vi "temperatureFGV.vi"(4 "error in (no error)":errorcluster, 5 "InputFan":bool=TRUE, 6 "state":T1, 7 "InputTemp":dbl) -> (0 "error out":errorcluster, 1 "OutputFan":bool=TRUE, 3 "OutputTemp":dbl)   [LabVIEW 2024]
uses:
  statesFGV.ctl
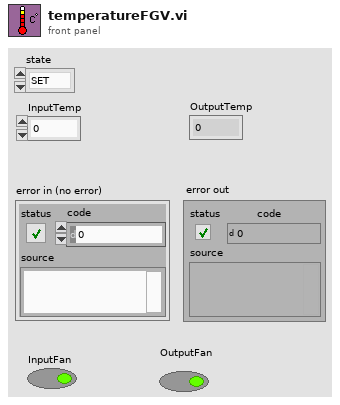
[diagram p1: front panel]
types:
  T1 = typedef "statesFGV.ctl" = enum16{"SET", "GET"}
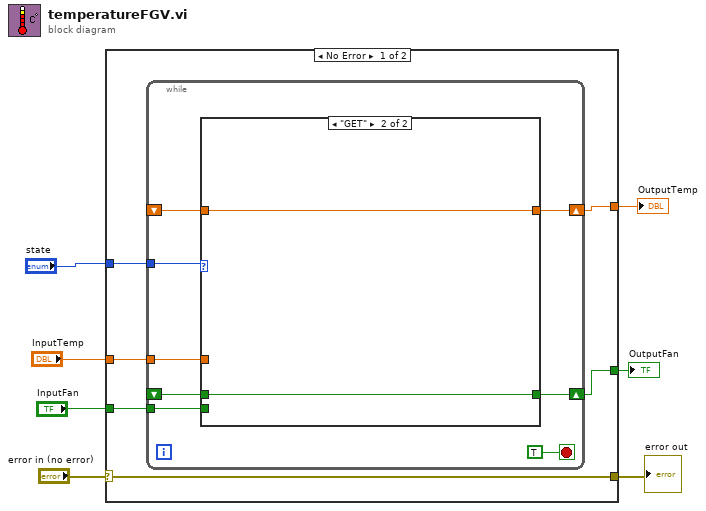
[diagram p0: block diagram]
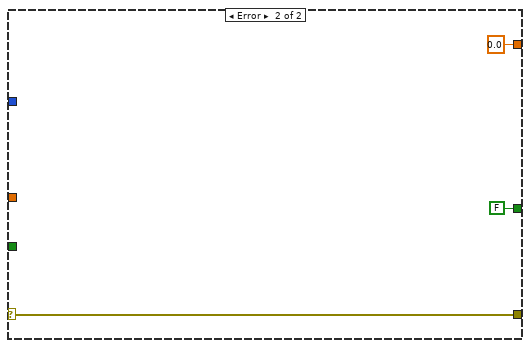
[diagram p3: hidden frame]
diagram:
  n1 = case shown="No Error" "error in (no error)" {
    selector: "error in (no error)" -> [w12 w28]
    tunnel: "state" -> [w13 _]
    tunnel: [w12 w28] -> w5
    tunnel: "InputTemp" -> [w11 _]
    tunnel: [w8 0.0 ("Input")] -> w3
    tunnel: "InputFan" -> [w10 _]
    tunnel: [w9 FALSE ("InputFan")] -> w1
    frame No Error {
      n2 = while {
        tunnel: w13 -> [w20]
        tunnel: w11 -> [w19]
        shift-right: [w18] -> w8
        shift-left: _ -> [w17]
        shift-right: [w15] -> w9
        shift-left: _ -> [w14]
        tunnel: w10 -> [w16]
        stop <- TRUE stop-if-true
        n3 = case shown="\"GET\"" w20 {
          tunnel: w19 -> [w22 _]
          tunnel: [w22 w25] -> w18
          tunnel: w17 -> [_ w25]
          tunnel: w16 -> [w23 _]
          tunnel: [w23 w24] -> w15
          tunnel: w14 -> [_ w24]
          frame "SET", Default {
          }
          frame "GET" {
          }
        }
      }
    }
    frame Error {
    }
  }
  "error out" <- w5
  "OutputTemp" <- w3
  "OutputFan" <- w1
